vi "Lesson3 - OR-gate wired to WHILE stop button.vi"() -> ()   [LabVIEW 2013]
panel:
  out "x*y":dbl
  in  "x":dbl
  in  "y":dbl
  in  "stop":bool
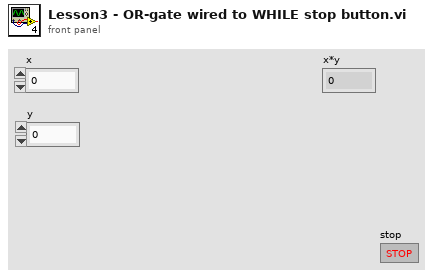
[diagram p1: front panel]
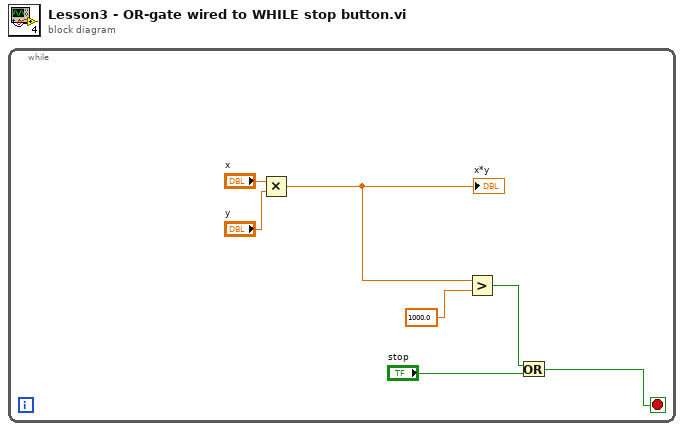
[diagram p0: block diagram]
diagram:
  n1 = while {
    stop <- w4 stop-if-true
    n2 = Multiply(x="x", y="y") -> (x*y=w3:dbl)
    "x*y" <- w3
    n3 = Greater?(x=w3, y=1000.0) -> (0:w1:bool)
    n4 = Or(x=w1, y="stop") -> (x .or. y?=w4:bool)
  }
